vi "ReadLime.vi"(1 "PathSuffix (0,1,2,none)":string) -> ()   [LabVIEW 2017]
uses:
  <vilib>/Rock Robotics/Network Tables/NT Read Number.vi
  Robot Global Data.vi
panel:
  out "Target":cluster{"x":dbl, "y":dbl, "A":dbl, "S":dbl}
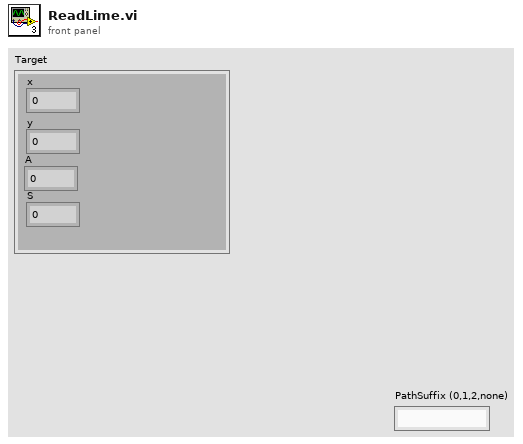
[diagram p1: front panel]
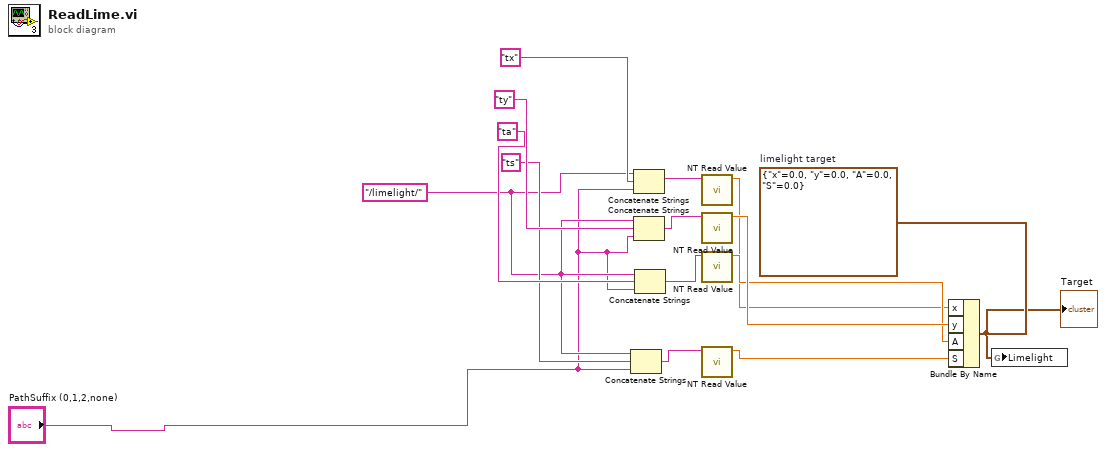
[diagram p0: block diagram]
diagram:
  w7 = "/limelight/"
  w16 = cluster{"x":dbl, "y":dbl, "A":dbl, "S":dbl} {"x"=0.0, "y"=0.0, "A"=0.0, "S"=0.0}  # limelight target
  n1 = Concatenate Strings(w7, "ts", "PathSuffix (0,1,2,none)") -> (w13:string)
  n2 = Concatenate Strings(w7, "tx", "PathSuffix (0,1,2,none)") -> (w15:string)
  n3 = Concatenate Strings(w7, "ty", "PathSuffix (0,1,2,none)") -> (w11:string)
  n4 = Concatenate Strings(w7, "ta", "PathSuffix (0,1,2,none)") -> (w12:string)
  n5 = call-poly <vilib>:"NT Read Value.vi"("Name"=w15) -> ("Numeric"=w3:dbl)  [unwired: 9 in, 1 out]
  n6 = call-poly <vilib>:"NT Read Value.vi"("Name"=w11) -> ("Numeric"=w6:dbl)  [unwired: 9 in, 1 out]
  n7 = call-poly <vilib>:"NT Read Value.vi"("Name"=w12) -> ("Numeric"=w5:dbl)  [unwired: 9 in, 1 out]
  n8 = call-poly <vilib>:"NT Read Value.vi"("Name"=w13) -> ("Numeric"=w2:dbl)  [unwired: 9 in, 1 out]
  n9 = Bundle By Name(cluster=w16, "x"=w3, "y"=w6, "A"=w5, "S"=w2) -> (w1:cluster{"x":dbl, "y":dbl, "A":dbl, "S":dbl})
  "Target" <- w1
  n10 = global write "Robot Global Data.vi" "Limelight"(w1) -> ()
